vi "t characterization spitball.vi"   [LabVIEW 2018]
uses:
  <vilib>/DAQmx/create/channels.llb/DAQmx Create Channel (AO-Voltage-Basic).vi
  <vilib>/DAQmx/create/channels.llb/DAQmx Create Channel (AI-Voltage-Basic).vi
  <vilib>/DAQmx/write.llb/DAQmx Write (Analog DBL 1Chan 1Samp).vi
  10e7368e-5fa8-467a-8f9e-f4c1b3e263ac.vi
  <vilib>/DAQmx/read.llb/DAQmx Read (Analog DBL 1Chan 1Samp).vi
  47650e4f-6bc4-4de2-8b0c-9520356e3e20.vi
types:
  T1 = cluster{"seconds since 1Jan1904":timestamp, "estimated polarization":dbl}[]
  T2 = cluster{"seconds since 1Jan1904":timestamp, "estimated polarization":dbl}
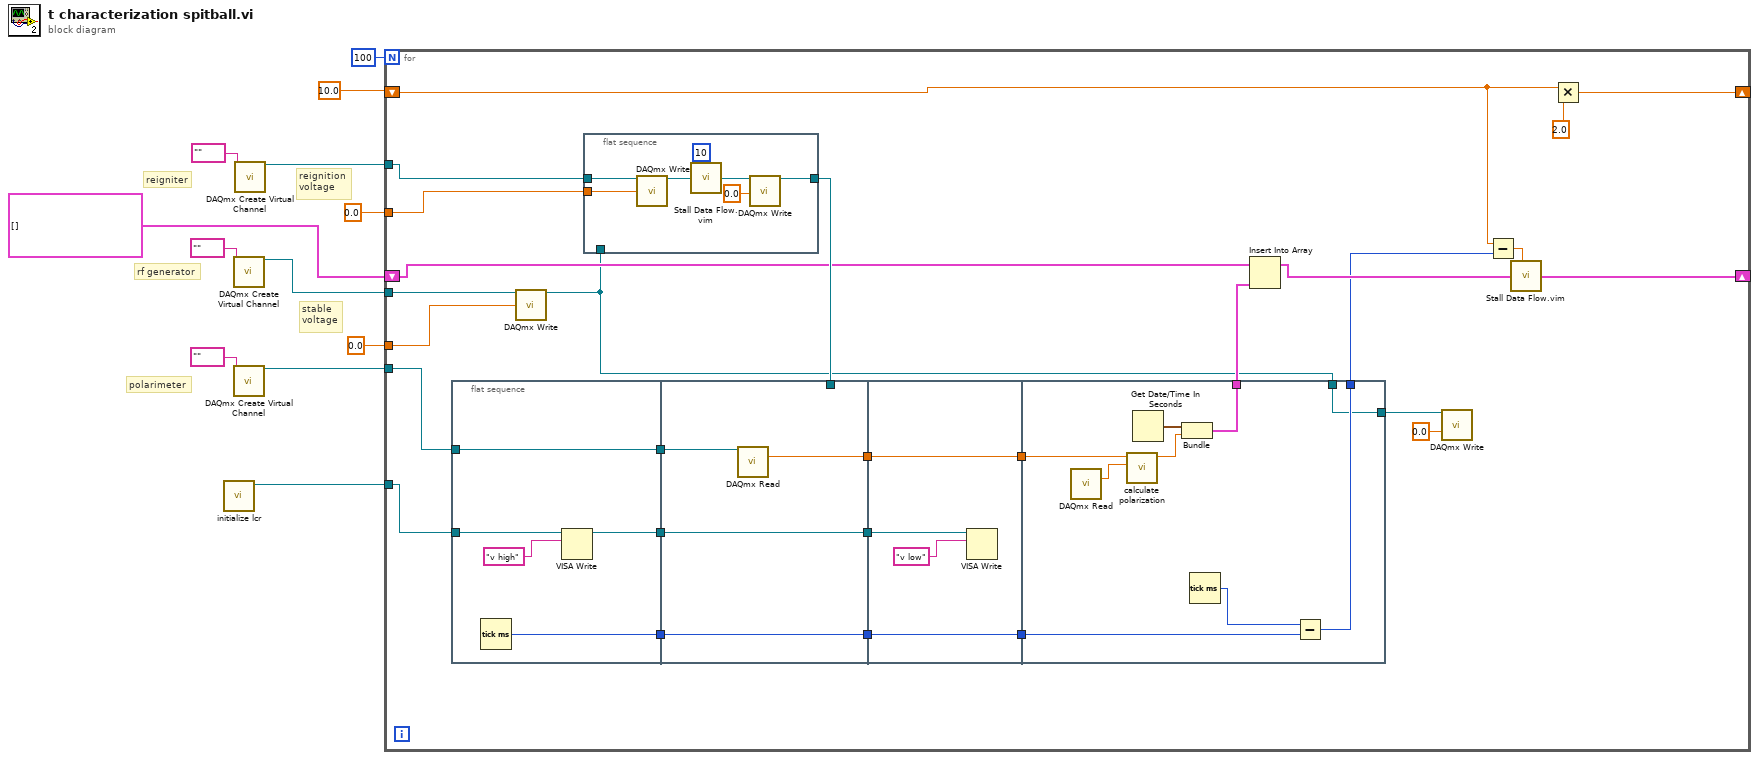
[diagram p0: block diagram]
diagram:
  # "stable\nvoltage"
  # "polarimeter"
  # "reignition\nvoltage"
  # "rf generator"
  # "reigniter"
  n1 = call "initialize lcr.vi"() -> ("VISA resource name out"=w6:refnum<visa-resource-name>)  [unwired: 11 in]
  n2 = call-poly <vilib>:"DAQmx Create Virtual Channel.vi"("physical channels"=tag "") -> ("task out"=w2:refnum<k21>)  [unwired: 13 in, 1 out]
  n3 = call-poly <vilib>:"DAQmx Create Virtual Channel.vi"("physical channels"=tag "") -> ("task out"=w7:refnum<k21>)  [unwired: 13 in, 1 out]
  n4 = call-poly <vilib>:"DAQmx Create Virtual Channel.vi"("physical channels"=tag "") -> ("task out"=w9:refnum<k21>)  [unwired: 13 in, 1 out]
  n5 = for {
    N: 100 -> [_]
    tunnel: w9 -> [w39]
    tunnel: 0.0 -> [w38]
    tunnel: w7 -> [w37]
    tunnel: w6 -> [w34]
    shift-right: [w24] -> _
    shift-left: T1 [] -> [w28]
    shift-right: [w26] -> _
    shift-left: 10.0 -> [w20]
    tunnel: w2 -> [w17]
    tunnel: 0.0 -> [w16]
    n6 = flat-sequence {
      tunnel: w37 -> [w51]
      tunnel: [w51] -> w35
      tunnel: w34 -> [w49]
      tunnel: [w48] -> w32
      tunnel: [w47] -> w21
      tunnel: w36 -> [_]
      tunnel: w35 -> [w55]
      tunnel: [w54] -> w33
      tunnel: w32 -> [w54]
      tunnel: [w53] -> w30
      tunnel: [w52] -> w22
      tunnel: w21 -> [w52]
      tunnel: w33 -> [w58]
      tunnel: [w57] -> w31
      tunnel: w30 -> [w57]
      tunnel: [w56] -> w23
      tunnel: w22 -> [w56]
      tunnel: w31 -> [w68]
      tunnel: [w64] -> w29
      tunnel: w23 -> [w62]
      tunnel: [w61] -> w19
      tunnel: w15 -> [w60]
      tunnel: [w60] -> w14
      frame #0 {
        n7 = Tick Count (ms)() -> (millisecond timer value=w47:u32)
        n8 = VISA Write(VISA resource name=w49, write buffer="v high") -> (VISA resource name out=w48:refnum<visa-resource-name>)  [unwired: 1 in, 2 out]
      }
      frame #1 {
        n9 = call-poly <vilib>:"DAQmx Read.vi"("task/channels in"=w55) -> ("data"=w53:dbl)  [unwired: 12 in, 2 out]
      }
      frame #2 {
        n10 = VISA Write(VISA resource name=w58, write buffer="v low") -> ()  [unwired: 1 in, 3 out]
      }
      frame #3 {
        n11 = call-poly <vilib>:"DAQmx Read.vi"() -> ("data"=w67:dbl)  [unwired: 13 in, 2 out]
        n12 = call "calculate polarization.vi"("min"=w67, "max"=w68) -> ("estimated polarization"=w65:dbl)  [unwired: 9 in]
        n13 = Get Date/Time In Seconds() -> (seconds since 1Jan1904=w66:timestamp)
        n14 = Bundle("seconds since 1Jan1904"=w66, "estimated polarization"=w65) -> (w64:T2)  [unwired: 1 in]
        n15 = Tick Count (ms)() -> (millisecond timer value=w63:u32)
        n16 = Subtract(x=w63, y=w62) -> (x-y=w61:u32)
      }
    }
    n17 = call-poly <vilib>:"DAQmx Write.vi"("task/channels in"=w17, "data"=w16) -> ("task out"=w15:refnum<k21>)  [unwired: 11 in, 2 out]
    n18 = flat-sequence {
      tunnel: w39 -> [w46]
      tunnel: w38 -> [w45]
      tunnel: [w41] -> w36
      tunnel: w15 -> [_]
      frame #0 {
        n19 = call-poly <vilib>:"DAQmx Write.vi"("task/channels in"=w46, "data"=w45) -> ("task out"=w42:refnum<k21>)  [unwired: 11 in, 2 out]
        n20 = call "Stall Data Flow.vim"("value in"=w42, "milliseconds to wait"=u32 10) -> ("value out"=w44:refnum<k21>)  [unwired: 1 out]
        n21 = call-poly <vilib>:"DAQmx Write.vi"("task/channels in"=w44, "data"=0.0) -> ("task out"=w41:refnum<k21>)  [unwired: 11 in, 2 out]
      }
    }
    n22 = Insert Into Array(array=w28, new element=w29) -> (w25:T1)  [unwired: 1 in]
    n23 = call-poly <vilib>:"DAQmx Write.vi"("task/channels in"=w14, "data"=0.0) -> ()  [unwired: 11 in, 3 out]
    n24 = Subtract(x=w20, y=w19) -> (x-y=w18:dbl)
    n25 = call "Stall Data Flow.vim"("value in"=w25, "milliseconds to wait"=w18) -> ("value out"=w24:T1)  [unwired: 1 out]
    n26 = Multiply(x=w20, y=2.0) -> (x*y=w26:dbl)
  }
